vi "Define Parameter.vi"(8 "error in (no error)":errorcluster, 11 "Analyze FF Spectrum in":refnum<class "Analyze FF Spectrum.lvclass">) -> (0 "error out":errorcluster, 3 "Analyze FF Spectrum out":refnum<class "Analyze FF Spectrum.lvclass">)   [LabVIEW 2020, in "Analyze.lvlib" / "Analyze FF Spectrum.lvclass"]
uses:
  Analyze FF Spectrum.lvclass
  Analyze Parameter/Analyze Parameter Spectral Calibration/Analyze Parameter Spectral Calibration.lvclass
  C:/POLARIS Programme/POLARIS-AS-3-Cams/Submodules/HIJ Vision/Analyze/Analyze Parameter/Analyze Parameter Base/Analyze Parameter Base.lvclass
  Analyze BaseClass/Analyze BaseClass/Analyze BaseClass.lvclass
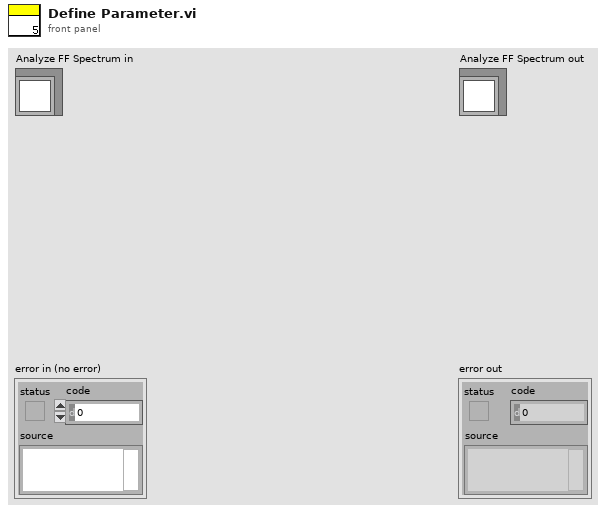
[diagram p1: front panel]
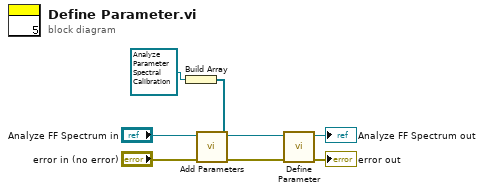
[diagram p0: block diagram]
diagram:
  n1 = Build Array(refnum<class "Analyze Parameter Spectral Calibration.lvclass"> refnum ("Spectral Calibration")) -> (w5:refnum<class "Analyze Parameter Spectral Calibration.lvclass">[])
  n2 = call-dynamic "Add Parameters.vi"("error in (no error)"="error in (no error)", "Parameters"=w5, "Analyze BaseClass in"="Analyze FF Spectrum in") -> ("error out"=w3:errorcluster, "Analyze BaseClass out"=w4:refnum<class "Analyze FF Spectrum.lvclass">)  [unwired: 7 in]
  n3 = call-parent "Define Parameter.vi"("error in (no error)"=w3, "Analyze BaseClass in"=w4) -> ("error out"=→"error out":errorcluster, "Analyze BaseClass out"=→"Analyze FF Spectrum out":refnum<class "Analyze FF Spectrum.lvclass">)  [unwired: 8 in]
